vi "Execute.vi"(8 "error in (no error)":errorcluster, 9 "System in":refnum<class "System.lvclass">, 10 "Command in":refnum<class "Command.lvclass">, 11 "CT-Stopping-State in":refnum<class "CT-Stopping-State.lvclass">) -> (0 "error out":errorcluster, 2 "Next State":refnum<class "State.lvclass">, 3 "CT-Stopping-State out":refnum<class "CT-Stopping-State.lvclass">)   [LabVIEW 2013, in "CT-Stopping-State.lvclass"]
uses:
  CT-Stopping-State.lvclass
  Commands/Command/Command.lvclass
  Systems/System/System.lvclass
  State/State.lvclass
  Systems/Catapult/Catapult.lvclass
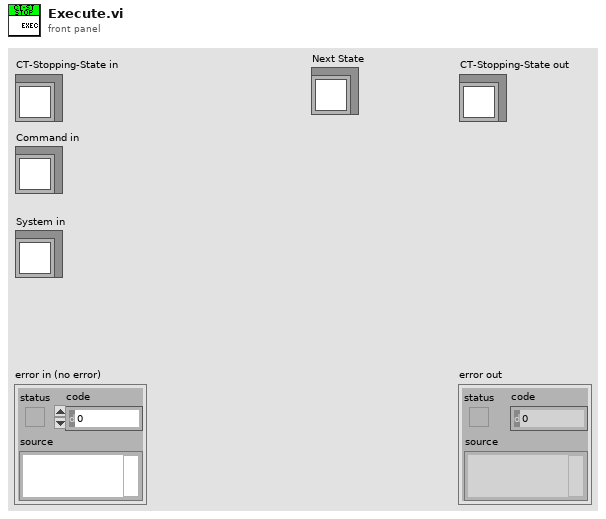
[diagram p1: front panel]
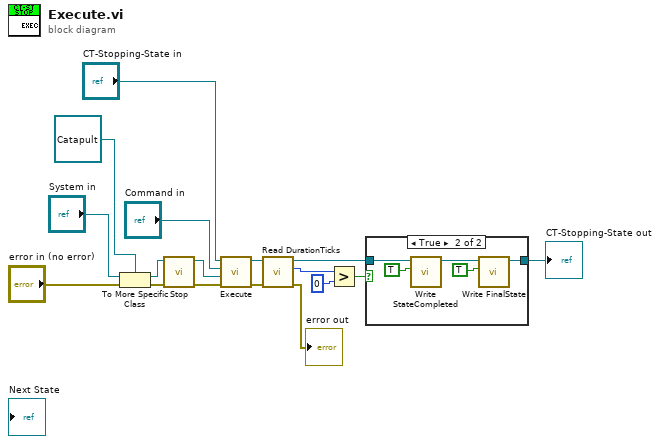
[diagram p0: block diagram]
diagram:
  n1 = To More Specific Class(target class=refnum<class "Catapult.lvclass"> refnum ("Catapult.lvclass"), reference="System in", error in="error in (no error)") -> (specific class reference=w12:refnum<class "Catapult.lvclass">, error out=w11:errorcluster)
  n2 = call-dynamic "Stop.vi"("error in (no error)"=w11, "Catapult in"=w12) -> ("error out"=w9:errorcluster, "Catapult out"=w10:refnum<class "Catapult.lvclass">)  [unwired: 8 in]
  n3 = call-parent "Execute.vi"("error in (no error)"=w9, "System in"=w10, "Command in"="Command in", "State in"="CT-Stopping-State in") -> ("error out"=w5:errorcluster, "State out"=w8:refnum<class "CT-Stopping-State.lvclass">)  [unwired: 5 in, 1 out]
  n4 = call "Read DurationTicks.vi"("error in (no error)"=w5, "State in"=w8) -> ("error out"=→"error out":errorcluster, "DurationTicks"=w7:u32, "State out"=w4:refnum<class "CT-Stopping-State.lvclass">)  [unwired: 7 in]
  n5 = Greater?(x=w7, y=u32 0) -> (0:w3:bool)
  n6 = case shown="True" w3 {
    tunnel: w4 -> [w18 w23]
    tunnel: [w18 w19] -> w2
    frame False {
    }
    frame True {
      n7 = call-dynamic "Write StateCompleted.vi"("StateCompleted"=TRUE, "State in"=w23) -> ("State out"=w20:refnum<class "CT-Stopping-State.lvclass">)  [unwired: 8 in, 1 out]
      n8 = call-dynamic "Write FinalState.vi"("FinalState"=TRUE, "State in"=w20) -> ("State out"=w19:refnum<class "CT-Stopping-State.lvclass">)  [unwired: 8 in, 1 out]
    }
  }
  "CT-Stopping-State out" <- w2
